vi "RSNRPZ Read Measurement.vi"(8 "error in (no error)":errorcluster, 9 "Timeout (5000 ms)":i32=5000, 10 "Channel (1)":i32=1, 11 "VISA session":refnum<visa-resource-name> caption="VISA resource name") -> (0 "error out":errorcluster, 2 "Measurement":dbl format="%.3p", 3 "dup VISA session":refnum<visa-resource-name> caption="VISA resource name")   [LabVIEW 2010]
doc: "This VI initiates an acquisition on the channels that you specifies in channel parameter. It then waits for the acquisition to complete, and returns the measurement for the channel you specify."
uses:
  rsnrpz_32.dll
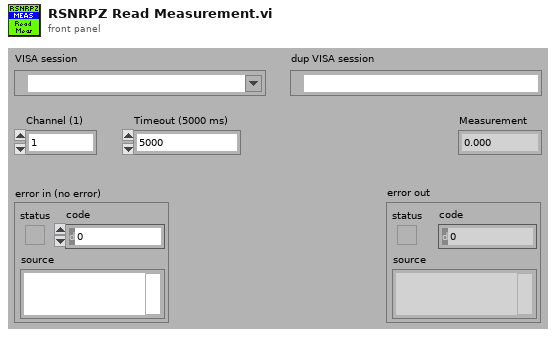
[diagram p1: front panel]
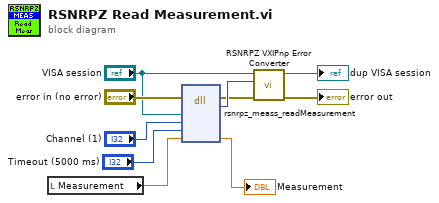
[diagram p0: block diagram]
diagram:
  n1 = local read "Measurement"() -> (w7:dbl)
  n2 = dll-call lib="rsnrpz_32.dll" fn="rsnrpz_meass_readMeasurement"(error in="error in (no error)", "Instrument Handle"="VISA session", "Channel"="Channel (1)", "Timeout (ms)"="Timeout (5000 ms)", "Measurement"=w7) -> (error out=w5:errorcluster, "Status"=w10:i32, "Measurement"=→"Measurement":dbl)  [unwired: 5 in, 1 out]
  n3 = call <instrlib>:"RSNRPZ VXIPnp Error Converter.vi"("error in"=w5, "VXIPnp error code"=w10, "VISA session"="VISA session") -> ("error out"=→"error out":errorcluster, "dup VISA session"=→"dup VISA session":refnum<visa-resource-name>)  [unwired: 7 in]
